vi "move_forward.vi"(5 "core_data in":T1) -> (0 "tour in progress":T3[](array[typedef]), 1 "chessboard":T4[][](array[typedef]), 2 "core_data out":T1)   [LabVIEW 2020, in "core.lvlib"]
uses:
  core.lvlib
  core_data/chess_square.ctl
  core_data/neighbour_square.ctl
  core_data/chessboard_index.ctl
  core_data/core_data.ctl
  core_data/tour_in_progress.ctl
  core_data/library_variable.vi
  core_data/core_data.lvlib
panel:
  # "Development\ncontrols/indicators useful for development and testing, but which are not outputs of the VI"
  # "Input\nInputs to the VI"
  # "Output\nOutputs of the VI"
  # "Description\n\nBlank VI with error handling case. \n\nSummarize the use of this VI in this space."
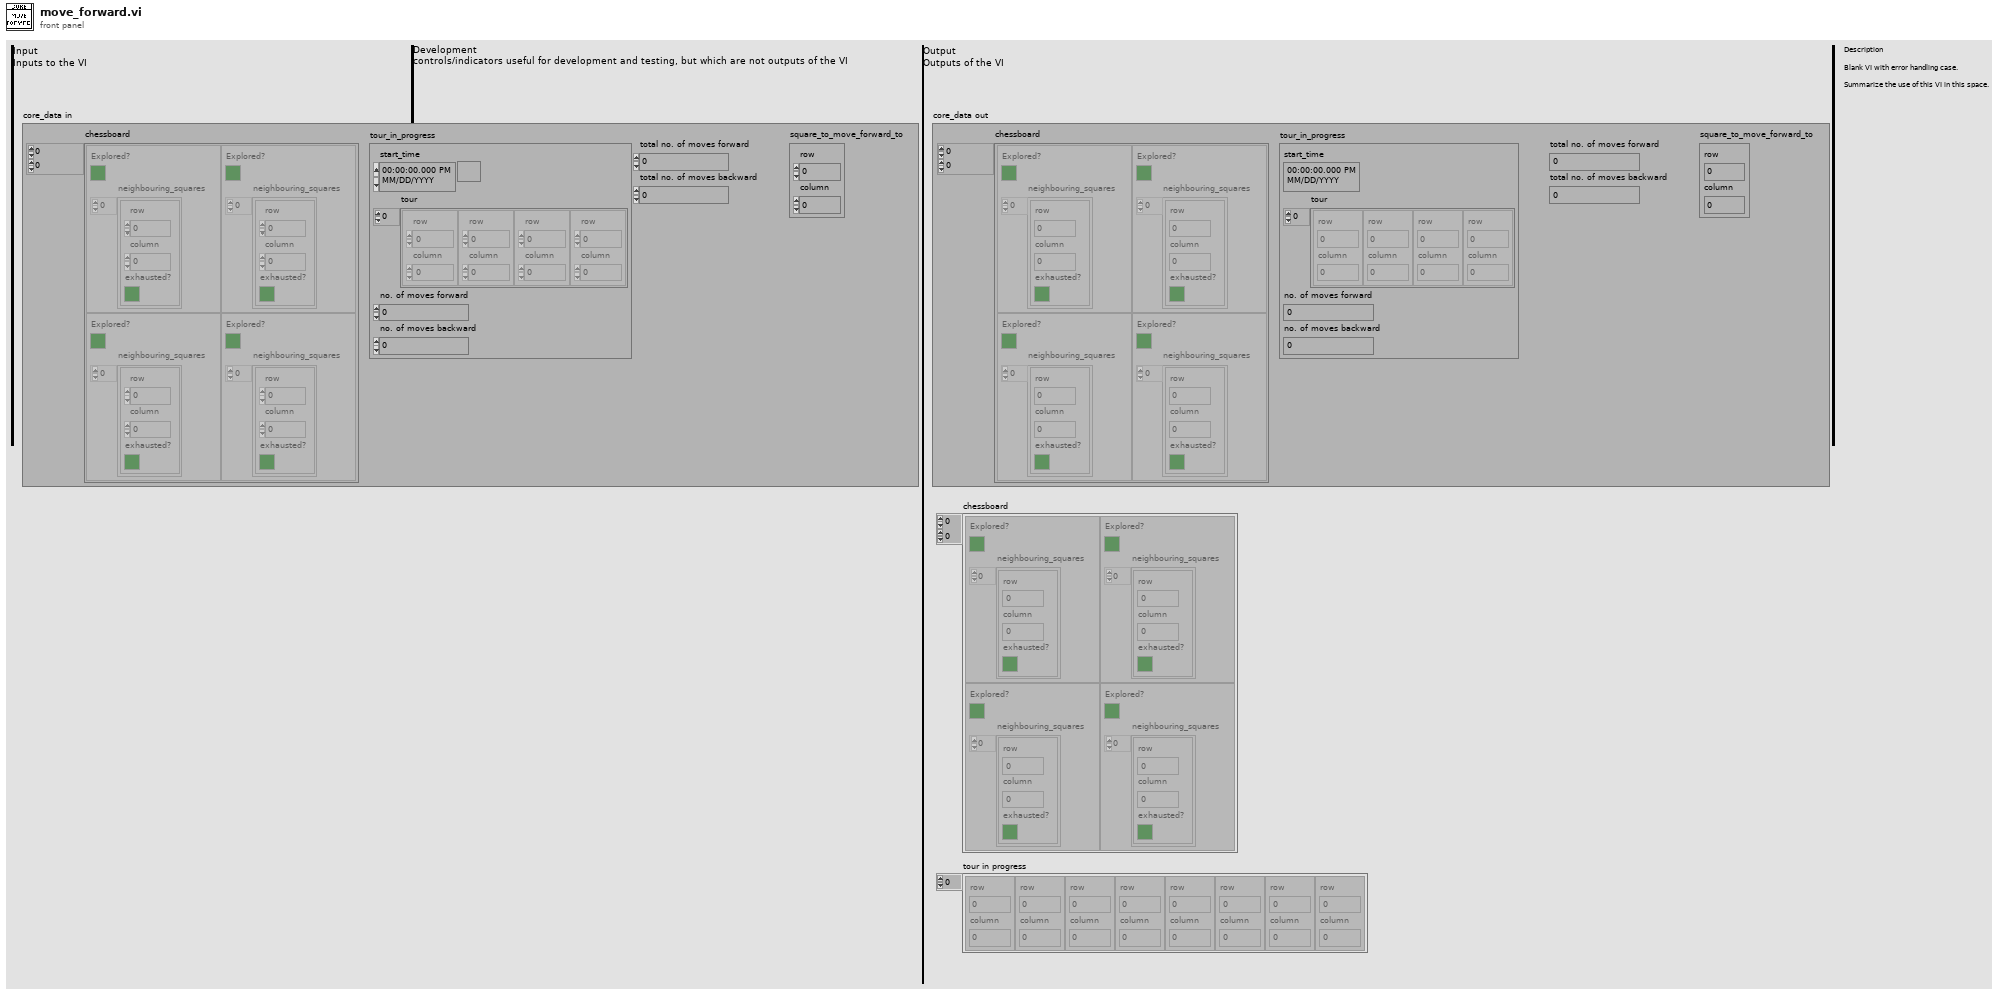
[diagram p1: front panel]
types:
  T1 = typedef "core.lvlib/core_data.lvlib/core_data.ctl" = cluster{"tour_in_progress":T2, "total no. of moves forward":u64, "total no. of moves backward":u64, "chessboard":T4[][], "square_to_move_forward_to":T3}
  T2 = typedef "core.lvlib/core_data.lvlib/tour_in_progress.ctl" = cluster{"start_time":timestamp, "tour":T3[], "no. of moves forward":u64, "no. of moves backward":u64}
  T3 = typedef "core.lvlib/core_data.lvlib/chessboard_index.ctl" = cluster{"row":u8, "column":u8}
  T4 = typedef "core.lvlib/core_data.lvlib/chess_square.ctl" = cluster{"Explored?":bool, "neighbouring_squares":T5[]}
  T5 = typedef "core.lvlib/core_data.lvlib/neighbour_square.ctl" = cluster{"row":u8, "column":u8, "exhausted?":bool}
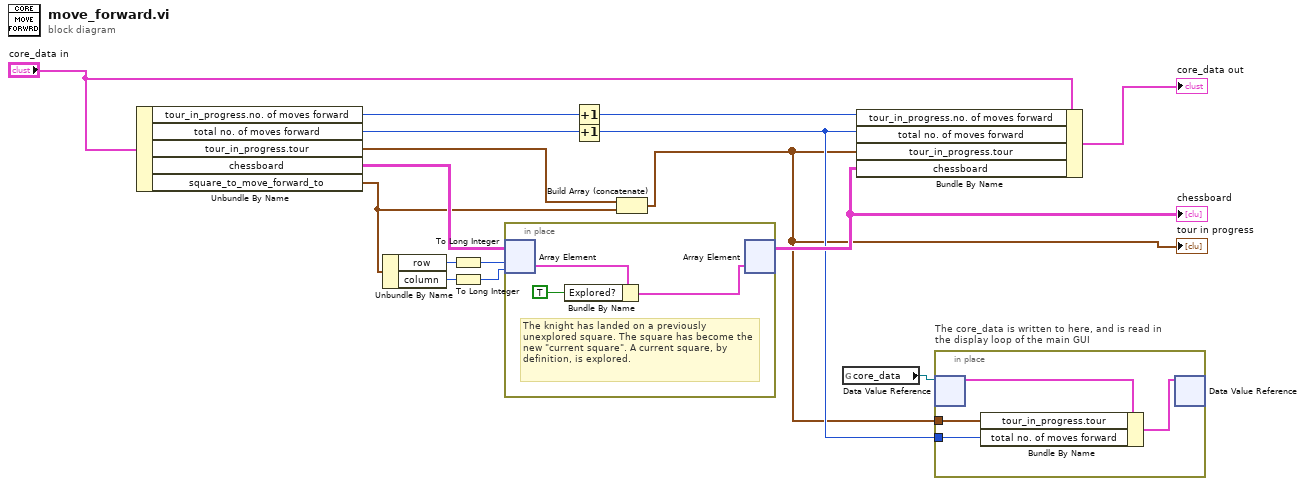
[diagram p0: block diagram]
diagram:
  n1 = Unbundle By Name("core_data in") -> ("tour_in_progress.no. of moves forward"=w8:u64, "total no. of moves forward"=w9:u64, "tour_in_progress.tour"=w15:T3[], "chessboard"=w14:T4[][], "square_to_move_forward_to"=w6:T3)
  n2 = Unbundle By Name(w6) -> ("row"=w13:u8, "column"=w12:u8)
  n3 = To Long Integer(number=w13) -> (32bit integer=w11:i32)
  n4 = To Long Integer(number=w12) -> (32bit integer=w10:i32)
  n5 = in-place {
    # "The knight has landed on a previously unexplored square. The square has become the new \"current square\". A current square, by definition, is explored."
    n6 = in-place-array #1(w14, w11, w10) -> (w19:T4)
    n7 = Bundle By Name(cluster=w19, "Explored?"=TRUE) -> (w17:T4)
    n8 = in-place-array #1(w17) -> (w16:T4[][])  [unwired: 2 out]
  }
  "chessboard" <- w16
  n9 = Increment(x=w8) -> (x+1=w7:u64)
  n10 = Increment(x=w9) -> (x+1=w3:u64)
  n11 = Build Array (concatenate)(w15, w6) -> (w1:T3[])
  "tour in progress" <- w1
  n12 = global read "library_variable.vi" "core_data"() -> (w2:refnum<data-value>)
  n13 = Bundle By Name(cluster="core_data in", "tour_in_progress.no. of moves forward"=w7, "total no. of moves forward"=w3, "tour_in_progress.tour"=w1, "chessboard"=w16) -> (→"core_data out":T1)
  n14 = in-place "The core_data is written to here, and is read in the display loop of the main GUI" {
    in-place-border: w1 -> [w21]
    in-place-border: w3 -> [w20]
    n15 = in-place-dvr #2(w2) -> (w23:T1)  [unwired: 1 out]
    n16 = Bundle By Name(cluster=w23, "tour_in_progress.tour"=w21, "total no. of moves forward"=w20) -> (w22:T1)
    n17 = in-place-dvr #2(w22) -> ()  [unwired: 2 out]
  }
